vi "Single Cam append frame_v1.2.vi"() -> ()   [LabVIEW 2024]
uses:
  <vilib>/vision/driver/NI_Vision_Acquisition_Software.lvlib
panel:
  in  "Analog Control::Gamma":dbl=0.800048828125 min=0.25 max=4.0 step=0.05
  in  "Analog Control::Black Level":dbl min=-5.0000011920928955 max=10.000002384185791
  in  "Analog Control::Gain":dbl min=0.0 max=27.045663671679687
  in  "Acquisition Control::Exposure Time":dbl=999.0 min=69.0 max=29999995.0
  in  "Stop (F)":bool
  in  "Frame rate":dbl
  out "Frames":i32
  out "Image":T1(plugin-control)
  out "Camera Information Array":T2(array[cluster]) {"BusType" format="%x"; "SerialNumberLow" format="%.0x"; "SerialNumberHigh" format="%.0x"}
  in  "Connected Only? (Yes)":bool=TRUE
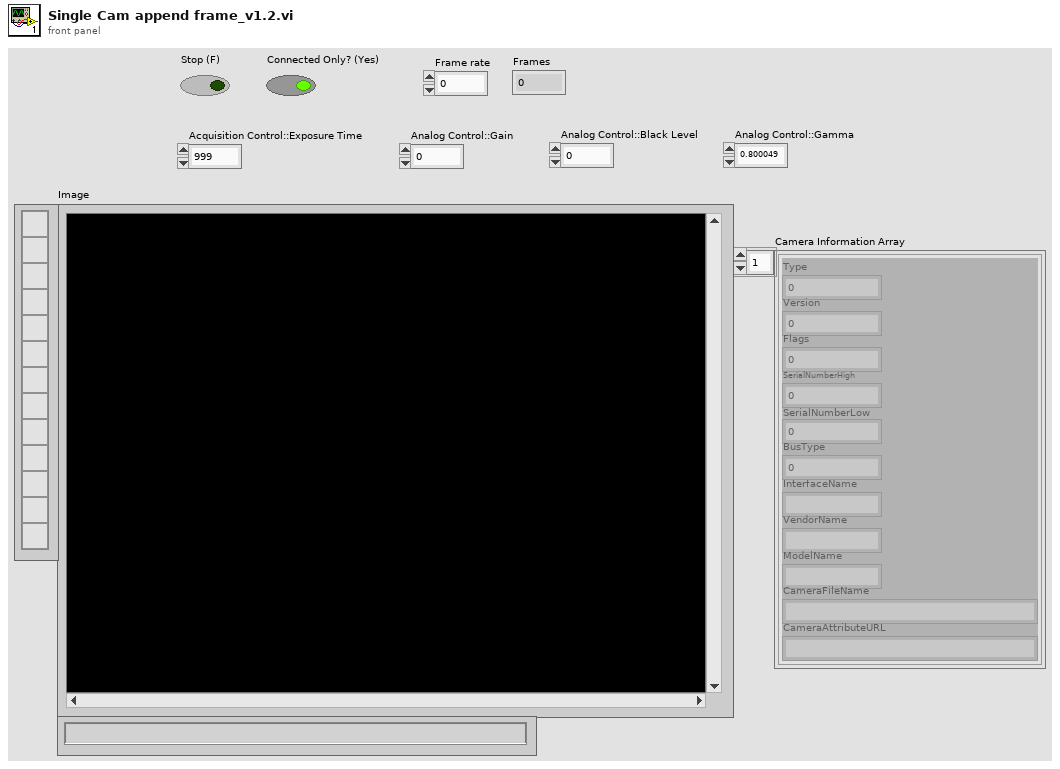
[diagram p1: front panel]
types:
  T1 = typedef "IMAQ Image.ctl" = refnum<image>
  T2 = cluster{"Type":u32, "Version":u32, "Flags":u32, "SerialNumberHigh":u32, "SerialNumberLow":u32, "BusType":u32, "InterfaceName":string, "VendorName":string, "ModelName":string, "CameraFileName":string, "CameraAttributeURL":string}[]
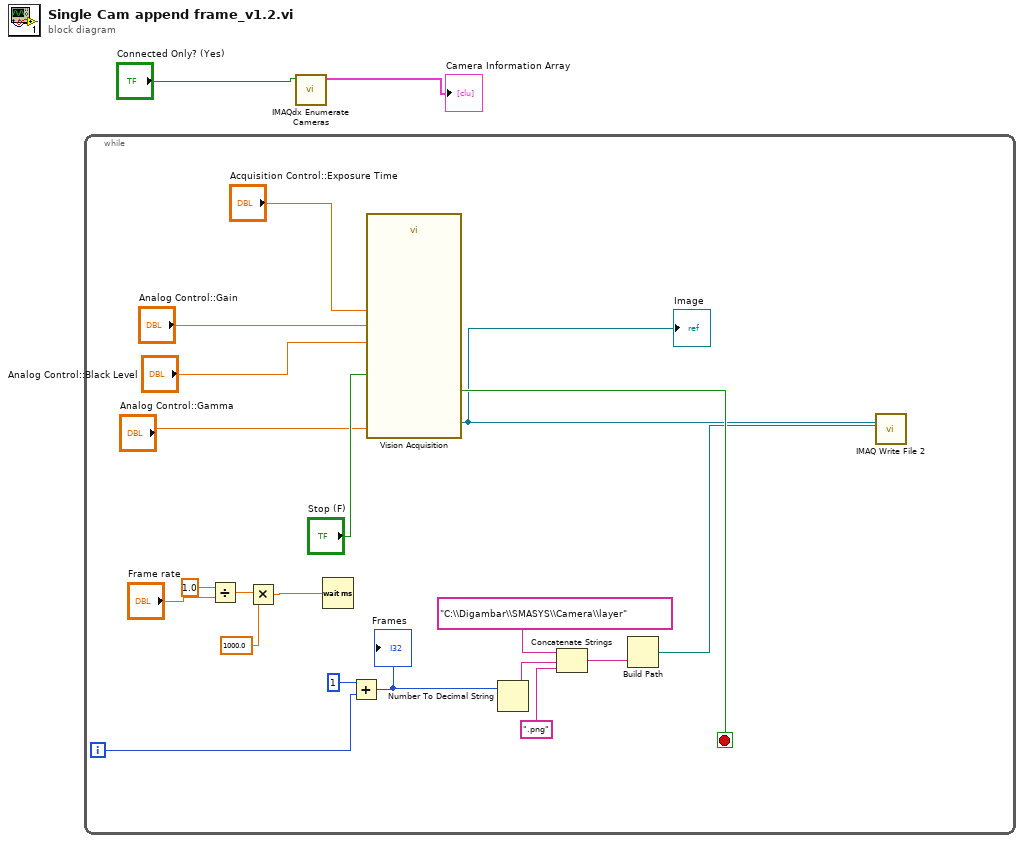
[diagram p0: block diagram]
diagram:
  n1 = while {
    i -> [w4]
    stop <- w21 stop-if-true
    n2 = Divide(x=1.0, y="Frame rate") -> (x/y=w9:dbl)
    n3 = Multiply(x=w9, y=1000.0) -> (x*y=w8:dbl)
    n4 = Wait (ms)(milliseconds to wait=w8) -> ()  [unwired: 1 out]
    n5 = Add(x=1, y=w4) -> (x+y=w15:i32)
    "Frames" <- w15
    n6 = call "Vision Acquisition"("Acquisition Control::Exposure Time"="Acquisition Control::Exposure Time", "Analog Control::Gain"="Analog Control::Gain", "Analog Control::Black Level"="Analog Control::Black Level", "Analog Control::Gamma"="Analog Control::Gamma", "Stop (F)"="Stop (F)") -> ("Image Out"=w20:T1, "Stopped"=w21:bool)  [unwired: 20 in, 1 out]
    "Image" <- w20
    n7 = Number To Decimal String(number=w15) -> (decimal integer string=w10:string)  [unwired: 1 in]
    n8 = Concatenate Strings("C:\\Digambar\\SMASYS\\Camera\\layer" ("string"), w10, ".png" ("string")) -> (w13:string)
    n9 = Build Path(name or relative path=w13) -> (appended path=w3:path)  [unwired: 1 in]
    n10 = call-poly "IMAQ Write File 2"("File Path"=w3, "Image"=w20) -> ()  [unwired: 8 in, 2 out]
  }
  n11 = call <vilib>:"IMAQdx Enumerate Cameras.vi"("Connected Only? (Yes)"="Connected Only? (Yes)") -> ("Camera Information Array"=→"Camera Information Array":T2)  [unwired: 9 in, 1 out]
